vi "NISE.remote.Get Property Enum Value Names.vi"(0 "SLSC Remote in":refnum<class "SLSC Interface.lvclass">, 5 "property":refnum<k21>, 11 "error in (no error)":errorcluster) -> (4 "SLSC Remote out":refnum<class "SLSC Interface.lvclass">, 6 "property out":refnum<k21>, 10 "Prop.Enum.ValueNames":string[](array[string]), 15 "error out":errorcluster)   [LabVIEW 2016, in "SLSC Interface.lvclass"]
uses:
  SLSC Interface Class/SLSC Interface.lvclass
  SLSC Interface Class/SLSC Interface.lvclass/SLSC Interface.ctl
  SLSC Interface Class/NISE.Read client handle.vi
  SLSC Interface Class/NISE.Read URL.vi
  SLSC Interface Class/NISE.Read session.vi
  <vilib>/httpClient/POSTBuffer.vi
  <vilib>/NI/JSON Support for LabVIEW/JSON Value/Object/Get Value/Get Value (Value).vi
  <vilib>/NI/JSON Support for LabVIEW/JSON Value/Array/Index Array/Index Array (String).vi
  <vilib>/httpClient/LabVIEWHTTPClient.lvlib
  <vilib>/NI/JSON Support for LabVIEW/JSON Value/JSON Value.lvclass
  <vilib>/NI/NI JSONRPC Server Framework/Classes/Client/JSONRPC Client.lvclass
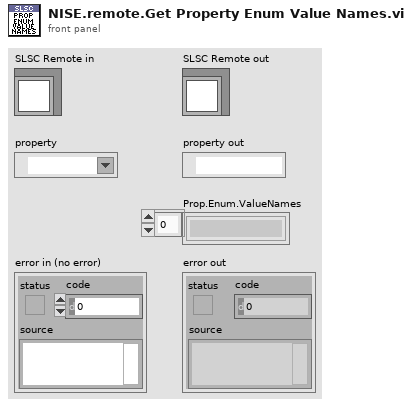
[diagram p1: front panel]
types:
  T1 = typedef "LabVIEWHTTPClient.lvlib/ClientHandle.ctl" = refnum<k1>
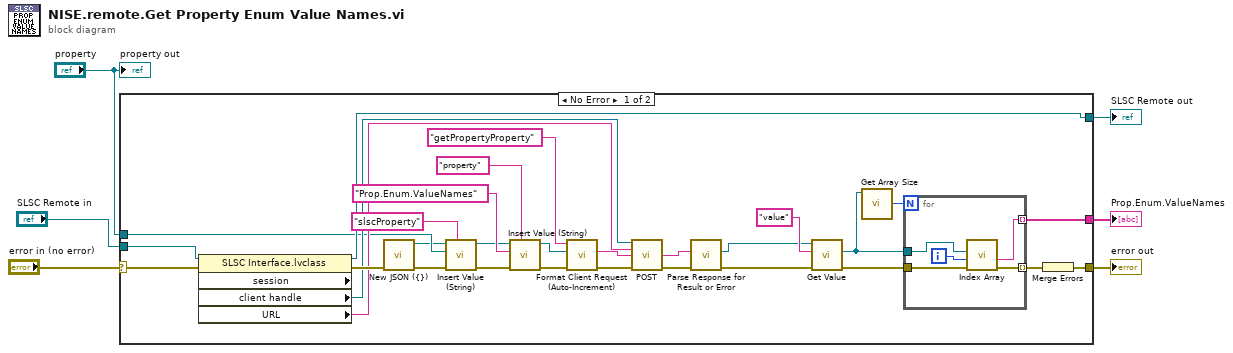
[diagram p0: block diagram]
diagram:
  n1 = case shown="No Error" "error in (no error)" {
    selector: "error in (no error)" -> [w34 w42]
    tunnel: "SLSC Remote in" -> [w36 w43]
    tunnel: [w35 w43] -> w4
    tunnel: [w15 w42] -> w1
    tunnel: [w16 _] -> w2
    tunnel: "property" -> [w14 _]
    frame No Error {
      n2 = property class="SLSC Interface.lvclass" props=["session", "client handle", "URL"](reference=w36, error in=w34) -> (reference out=w35:refnum<class "SLSC Interface.lvclass">, error out=w33:errorcluster, "client handle"=w29:T1, "URL"=w28:string)  [unwired: 1 out]
      n3 = call <vilib>:"New JSON ({}).vi"("error in (no error)"=w33) -> ("error out"=w32:errorcluster, "JSON Value out"=w12:refnum<class "JSON Value.lvclass">)  [unwired: 9 in]
      n4 = call <vilib>:"Insert Value (String).vi"("key"="slscProperty" ("Name"), "error in (no error)"=w32, "value"=w14, "JSON Value in"=w12) -> ("error out"=w22:errorcluster, "JSON Value out"=w11:refnum<class "JSON Value.lvclass">)  [unwired: 5 in, 1 out]
      n5 = call <vilib>:"Insert Value (String).vi"("key"="property" ("Name"), "error in (no error)"=w22, "value"="Prop.Enum.ValueNames" ("String"), "JSON Value in"=w11) -> ("error out"=w23:errorcluster, "JSON Value out"=w24:refnum<class "JSON Value.lvclass">)  [unwired: 5 in, 1 out]
      n6 = call <vilib>:"Format Client Request (Auto-Increment).vi"("error in (no error)"=w23, "JSON Value in"=w24, "method"="getPropertyProperty") -> ("error out"=w27:errorcluster, "Request String"=w30:string)  [unwired: 7 in]
      n7 = call-poly <vilib>:"POST.vi"("client handle"=w29, "url"=w28, "buffer"=w30, "error in (no error)"=w27) -> ("body"=w26:string, "error out"=w25:errorcluster)  [unwired: 8 in, 2 out]
      n8 = call <vilib>:"Parse Response for Result or Error.vi"("error in"=w25, "Response String In"=w26) -> ("error out"=w8:errorcluster, "JSON Value out"=w7:refnum<class "JSON Value.lvclass">)  [unwired: 7 in, 1 out]
      n9 = call-poly <vilib>:"Get Value.vi"("error in (no error)"=w8, "key"="value" ("Parameter Name"), "JSON Value in"=w7) -> ("error out"=w18:errorcluster, "JSON Value out"=w19:refnum<class "JSON Value.lvclass">)  [unwired: 7 in]
      n10 = call <vilib>:"Get Array Size.vi"("JSON Value in"=w19) -> ("size(s)"=w20:i32)  [unwired: 9 in, 1 out]
      n11 = for {
        N: w20 -> [_]
        tunnel: w19 -> [w40]
        tunnel: w18 -> [w39]
        tunnel: [w38] -> w17 mode=indexing
        tunnel: [w37] -> w16 mode=indexing
        i -> [w41]
        n12 = call-poly <vilib>:"Index Array.vi"("error in (no error)"=w39, "index"=w41, "JSON Value in"=w40) -> ("error out"=w38:errorcluster, "String"=w37:string)  [unwired: 7 in]
      }
      n13 = Merge Errors(w17) -> (w15:errorcluster)
    }
    frame Error {
    }
  }
  "error out" <- w1
  "SLSC Remote out" <- w4
  "Prop.Enum.ValueNames" <- w2
  "property out" <- "property"
